vi "Calculate spiral radii for current iteration.vi"(0 "Number of spirals":u32, 1 "Start radius (V)":dbl, 2 "End radius (V)":dbl, 3 "Run pattern":bool, 4 "Time between post-bleaching\ngates (ms)":u32) -> (5 "Radius 1":dbl, 6 "Radius 2":dbl, 8 "Spirals completed?":bool)   [LabVIEW 2011]
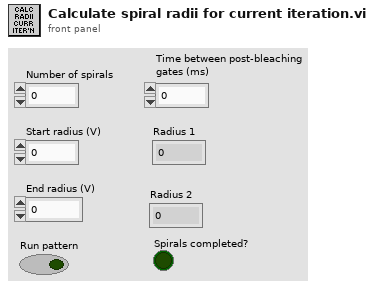
[diagram p1: front panel]
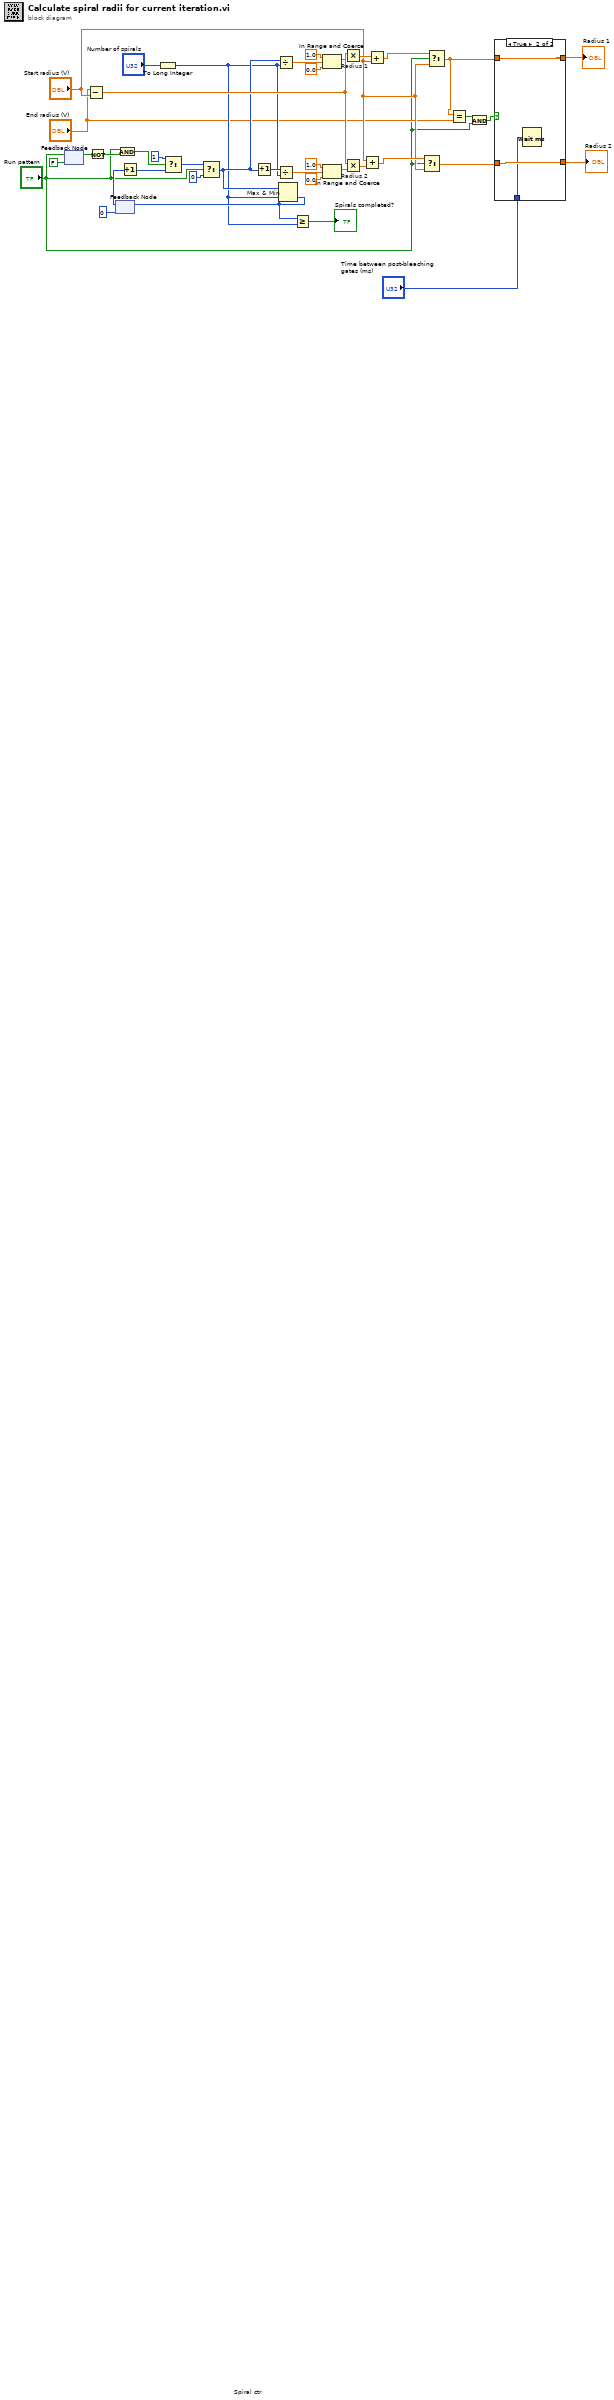
[diagram p0: block diagram]
diagram:
  n1 = feedback #1(FALSE ("Start pattern")) -> (w20:bool)
  n2 = feedback-in #1("Run pattern") -> ()
  n3 = Subtract(x="End radius (V)", y="Start radius (V)") -> (x-y=w38:dbl)
  n4 = Not(x=w20) -> (.not. x?=w21:bool)
  n5 = feedback #2 "Spiral ctr"(0) -> (w25:i32)
  n6 = And(x="Run pattern", y=w21) -> (x .and. y?=w22:bool)
  n7 = Increment(x=w25) -> (x+1=w26:i32)
  n8 = To Long Integer(number="Number of spirals") -> (32bit integer=w14:i32)
  n9 = Select(t=1, s=w22, f=w26) -> (s? t:f=w27:i32)
  n10 = Select(t=w27, s="Run pattern", f=0) -> (s? t:f=w36:i32)
  n11 = Increment(x=w36) -> (x+1=w15:i32)
  n12 = Divide(x=w36, y=w14) -> (x/y=w32:dbl)
  n13 = Divide(x=w15, y=w14) -> (x/y=w28:dbl)
  n14 = Max & Min(x=w36, y=w14) -> (min(x,y)=w17:i32)  [unwired: 1 out]
  n15 = feedback-in #2(w17) -> ()
  n16 = Greater Or Equal?(x=w17, y=w14) -> (x >= y?=→"Spirals completed?":bool)
  n17 = In Range and Coerce(upper limit=1.0, x=w32, lower limit=0.0) -> (coerced(x)=w34:dbl)  [unwired: 1 out]
  n18 = In Range and Coerce(upper limit=1.0, x=w28, lower limit=0.0) -> (coerced(x)=w31:dbl)  [unwired: 1 out]
  n19 = Multiply "Radius 1"(x=w38, y=w34) -> (x*y=w13:dbl)
  n20 = Multiply "Radius 2"(x=w38, y=w31) -> (x*y=w39:dbl)
  n21 = Add(x="Start radius (V)", y=w39) -> (x+y=w11:dbl)
  n22 = Add(x=w13, y="Start radius (V)") -> (x+y=w12:dbl)
  n23 = Select(t=w11, s="Run pattern", f="Start radius (V)") -> (s? t:f=w7:dbl)
  n24 = Select(t=w12, s="Run pattern", f="Start radius (V)") -> (s? t:f=w6:dbl)
  n25 = Equal?(x=w6, y="End radius (V)") -> (x = y?=w4:bool)
  n26 = And(x=w4, y="Run pattern") -> (x .and. y?=w2:bool)
  n27 = case shown="True" w2 {
    tunnel: [w41 w44] -> w9
    tunnel: w6 -> [w41 w44]
    tunnel: [w40 w43] -> w8
    tunnel: w7 -> [w40 w43]
    tunnel: "Time between post-bleaching\ngates (ms)" -> [_ w42]
    frame False {
    }
    frame True {
      n28 = Wait (ms)(milliseconds to wait=w42) -> ()  [unwired: 1 out]
    }
  }
  "Radius 2" <- w8
  "Radius 1" <- w9
